vi "subvi_write_motor_direction.vi"(9 "Current Angles":cluster{"Analyser 1":i32, "Analyser 2":i32}, 10 "Set Angles":cluster{"Analyser 1":i32, "Analyser 2":i32}, 11 "Analysers Moving?":T1) -> (0 "Directions":cluster{"Analyser 1":bool, "Analyser 2":bool}, 3 "Analysers Moving? Output":T1)   [LabVIEW 2014]
doc: "Sub VI to write to the analyser motors the direction they are set to move in and returns\nthe direction bools as a cluster.\nManish Patel\nLast date edited: 15/08/2019"
panel:
  # "INPUTS"
  # "OUTPUTS"
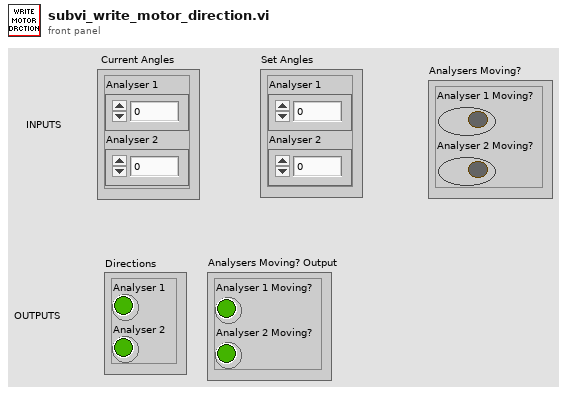
[diagram p1: front panel]
types:
  T1 = cluster{"Analyser 1 Moving?":bool, "Analyser 2 Moving?":bool}
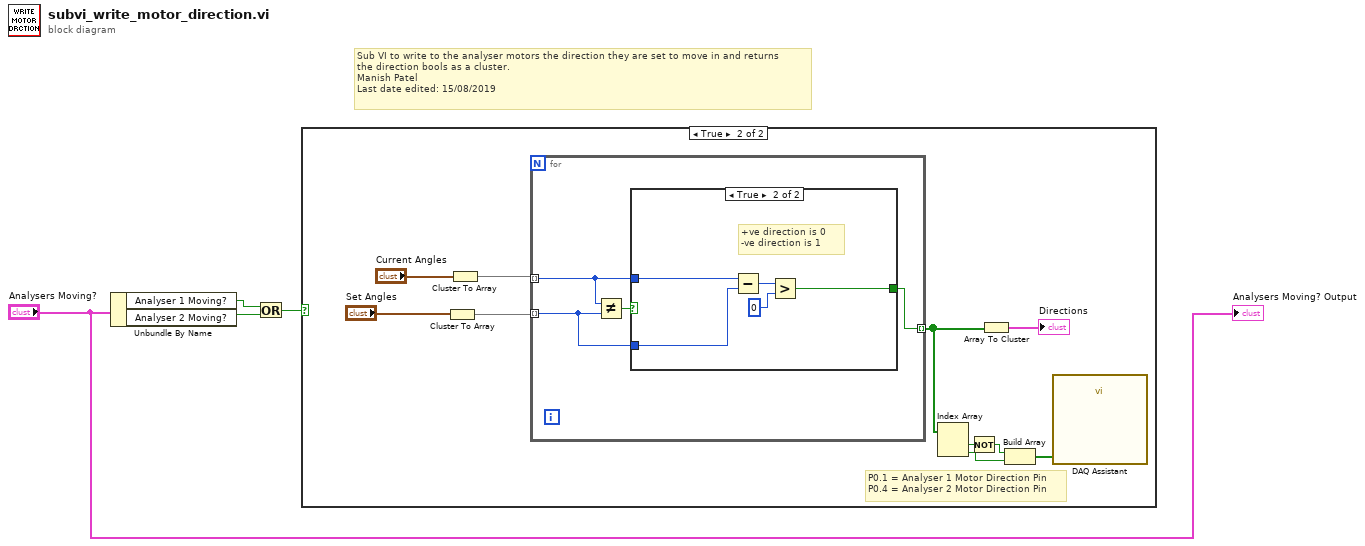
[diagram p0: block diagram]
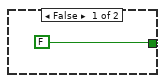
[diagram p3: hidden frame]
diagram:
  # "Sub VI to write to the analyser motors the direction they are set to move in and returns\nthe direction bools as a cluster.\nManish Patel\nLast date edited: 15/08/2019"
  n1 = Unbundle By Name("Analysers Moving?") -> ("Analyser 1 Moving?"=w2:bool, "Analyser 2 Moving?"=w1:bool)
  n2 = Or(x=w2, y=w1) -> (x .or. y?=w3:bool)
  n3 = case shown="True" w3 {
    frame False {
    }
    frame True {
      # "P0.1 = Analyser 1 Motor Direction Pin\nP0.4 = Analyser 2 Motor Direction Pin"
      n4 = Cluster To Array(cluster="Set Angles") -> (array=w11:i32[])
      n5 = Cluster To Array(cluster="Current Angles") -> (array=w12:i32[])
      n6 = for {
        tunnel: w11 -> [w16] mode=indexing
        tunnel: w12 -> [w17] mode=indexing
        tunnel: [w15] -> w7 mode=indexing
        n7 = Not Equal?(x=w17, y=w16) -> (x != y?=w18:bool)
        n8 = case shown="True" w18 {
          tunnel: w17 -> [_ w21]
          tunnel: w16 -> [_ w20]
          tunnel: [FALSE w22] -> w15
          frame False {
          }
          frame True {
            # "+ve direction is 0\n-ve direction is 1"
            n9 = Subtract(x=w21, y=w20) -> (x-y=w24:i32)
            n10 = Greater?(x=w24, y=0) -> (0:w22:bool)
          }
        }
      }
      n11 = Index Array(array=w7) -> (element #1=w8:bool, element #2=w6:bool)  [unwired: 2 in]
      n12 = Not(x=w8) -> (.not. x?=w9:bool)
      n13 = Array To Cluster(array=w7) -> (cluster=→"Directions":cluster{"[0]":bool, "[1]":bool})
      n14 = Build Array(w9, w6) -> (w5:bool[])
      n15 = call "DAQ Assistant"("data"=w5) -> ()  [unwired: 17 in, 2 out]
    }
  }
  "Analysers Moving? Output" <- "Analysers Moving?"
